vi "Fit_2D_Gauss.vi"(0 "Enum":enum16{"Gauss", "Lorentz"}(ring), 7 "Image IN":dbl[][](array[numeric])) -> (8 "Fit Parameters":dbl[](array[numeric]), 10 "Fit Image":dbl[][](array[numeric]))   [LabVIEW 2014]
uses:
  <vilib>/gmath/NumericalOptimization/Nonlinear Curve Fit LM.vi
  <vilib>/gmath/NI_Gmath.lvlib
panel:
  in  "termination":cluster{"max iteration":i32, "tolerance":dbl}={"max iteration"=40, "tolerance"=1e-08}
  out "residue":dbl
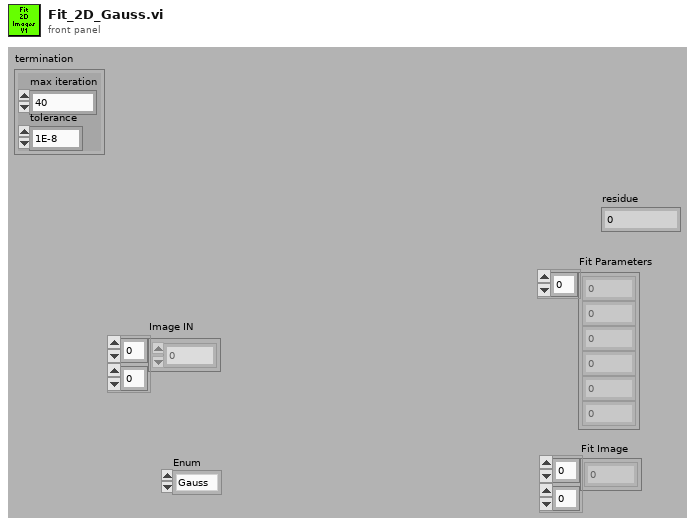
[diagram p1: front panel]
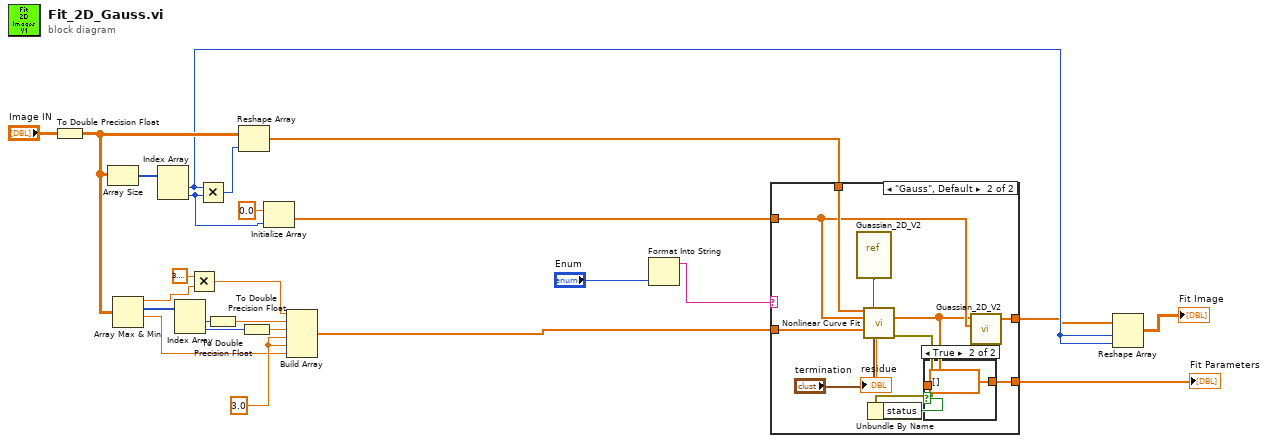
[diagram p0: block diagram]
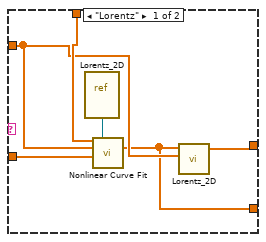
[diagram p2: hidden frame]
diagram:
  w2 = 3.0 ("element")
  n1 = To Double Precision Float(number="Image IN") -> (double precision float=w13:dbl[][])
  n2 = Array Size(array=w13) -> (size(s)=w22:i32[])
  n3 = Array Max & Min(array=w13) -> (max value=w12:dbl, max index (indices)=w18:i32[], min value=w1:dbl)  [unwired: 1 out]
  n4 = Index Array(array=w22) -> (element #1=w7:i32, element #2=w10:i32)  [unwired: 2 in]
  n5 = Index Array(array=w18) -> (element #1=w15:i32, element #2=w14:i32)  [unwired: 2 in]
  n6 = Multiply(x=3.141592653589793, y=w12) -> (x*y=w19:dbl)
  n7 = Multiply(x=w7, y=w10) -> (x*y=w21:i32)
  n8 = To Double Precision Float(number=w15) -> (double precision float=w17:dbl)
  n9 = Reshape Array(w13, w21) -> (w9:dbl[])
  n10 = To Double Precision Float(number=w14) -> (double precision float=w16:dbl)
  n11 = Initialize Array(0.0 ("element"), w10) -> (w8:dbl[])
  n12 = Build Array(w19, w17, w16, w2, w2, w1) -> (w5:dbl[])
  n13 = Format Into String("Enum") -> (resulting string=w3:string)  [unwired: 3 in, 1 out]
  n14 = case shown="\"Gauss\", Default" w3 {
    tunnel: [w26 w32] -> w25
    tunnel: w9 -> [w29 w41]
    tunnel: w8 -> [w28 w40]
    tunnel: [w27 w39] -> w6
    tunnel: w5 -> [w30 w38]
    frame "Lorentz" {
      n15 = vi-ref "Lorentz_2D.vi"() -> (w31:refnum<vi>)
      n16 = call-poly <vilib>:"Nonlinear Curve Fit.vi"("Y"=w29, "f(x,a)"=w31, "X"=w28, "initial parameters"=w30) -> ("best fit parameters"=w26:dbl[])  [unwired: 6 in, 5 out]
      n17 = call "Lorentz_2D.vi"("X"=w28, "a"=w26) -> ("f(X,a)"=w27:dbl[])  [unwired: 2 in, 2 out]
    }
    frame "Gauss", Default {
      n18 = vi-ref "Guassian_2D_V2.vi"() -> (w42:refnum<vi>)
      n19 = call-poly <vilib>:"Nonlinear Curve Fit.vi"("Y"=w41, "f(x,a)"=w42, "X"=w40, "initial parameters"=w38, "termination"="termination") -> ("best fit parameters"=w33:dbl[], "residue"=→"residue":dbl, "error out"=w35:errorcluster)  [unwired: 5 in, 3 out]
      n20 = Unbundle By Name(w35) -> ("status"=w34:bool)
      n21 = case shown="True" w34 {
        tunnel: w33 -> [w43 _]
        tunnel: [w43 dbl[] [] ("best fit parameters")] -> w32
        frame False {
        }
        frame True {
        }
      }
      n22 = call "Guassian_2D_V2.vi"("X"=w40, "a"=w33) -> ("f(X,a)"=w39:dbl[])  [unwired: 2 in, 2 out]
    }
  }
  "Fit Parameters" <- w25
  n23 = Reshape Array(w6, w7, w7) -> (→"Fit Image":dbl[][])
